vi "Remove From SubPanel.vi"(8 "Error In":errorcluster, 11 "Display Panel V3 in":refnum<class "Display Panel V3.lvclass">) -> (0 "Error Out":errorcluster, 3 "Display Panel V3 out":refnum<class "Display Panel V3.lvclass">)   [LabVIEW 2014, in "Display Panel.lvlib" / "Display Panel V3.lvclass"]
uses:
  Display Panel V3.lvclass
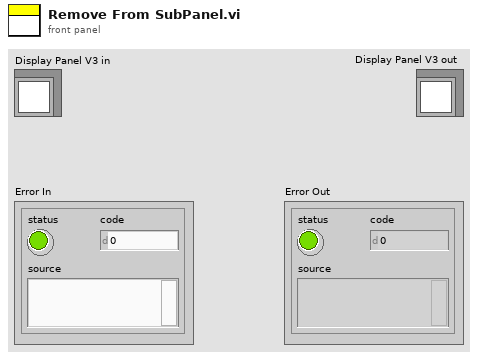
[diagram p1: front panel]
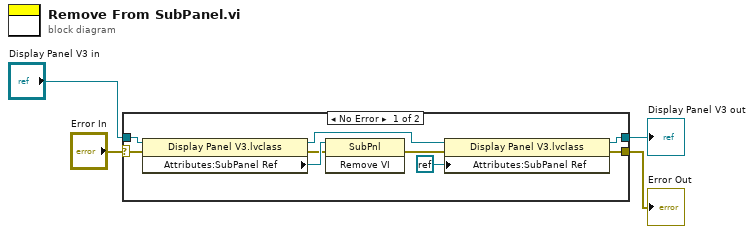
[diagram p0: block diagram]
diagram:
  n1 = case shown="No Error" "Error In" {
    selector: "Error In" -> [w5 w14]
    tunnel: "Display Panel V3 in" -> [w13 w15]
    tunnel: [w7 w15] -> w2
    tunnel: [w6 w14] -> w1
    frame No Error {
      n2 = property class="Display Panel V3.lvclass"(reference=w13, error in=w5) -> (reference out=w10:refnum<class "Display Panel V3.lvclass">, error out=w11:errorcluster, "Attributes:SubPanel Ref"=w12:refnum<vi>)
      n3 = invoke class="SubPnl" method="Remove VI"(reference=w12, error in=w11) -> (error out=w9:errorcluster)  [unwired: 1 in, 2 out]
      n4 = property class="Display Panel V3.lvclass"(reference=w10, error in=w9, "Attributes:SubPanel Ref"=refnum<k0> refnum) -> (reference out=w7:refnum<class "Display Panel V3.lvclass">, error out=w6:errorcluster)
    }
    frame Error {
    }
  }
  "Display Panel V3 out" <- w2
  "Error Out" <- w1
